vi "流量计UI.vi"() -> ()   [LabVIEW 2016]
uses:
  <vilib>/Plasmionique/MB Master/MB_Master_Serial/MB_Master_Serial.lvclass
  D:/Program Files (x86)/National Instruments/LabVIEW 2016/vi.lib/Plasmionique/MB Master/MB_Master/MB_Master.lvclass
  <vilib>/Analysis/baseanly.llb/Mean (DBL).vi
  <vilib>/Utility/config.llb/NI_LVConfig.lvlib
  <vilib>/Analysis/NI_AALBase.lvlib
panel:
  out "水位":dbl
  out "累积流量":dbl
  out "瞬时流速":dbl
  out "瞬时流量":dbl
  in  "选项卡控件":enum32{"LDM51", "MGG/KL QC", "斯坦道功率测流"}(tab)
  out "数组":T1[](array[typedef])
  out "数组 2":T2[](array[typedef]) {"累积流量单位" items=["L", "M3", "T", "USG"]; "瞬时流量单位" items=["L/S", "L/M", "L/H", "M3/S", "M3/M", "M3/H", "T/S", "T/M", "T/H", "GPS", "GPM", "GPH"]}
  out "数组 3":T5[](array[typedef])
  out "MB_Serial session":refnum<class "MB_Master_Serial.lvclass">
  in  "斯坦道功率测流":bool
  in  "流量计启用 3":bool
  in  "数量 3":u16
  out "流量计类型 3":T6=enum."斯坦道功率测流"
  in  "流量计启用 2":bool
  in  "数量 2":u16
  out "流量计类型 2":T6=enum."MGG/KL QC"
  in  "数量":u16
  out "流量计类型":T6
  in  "流量计启用":bool
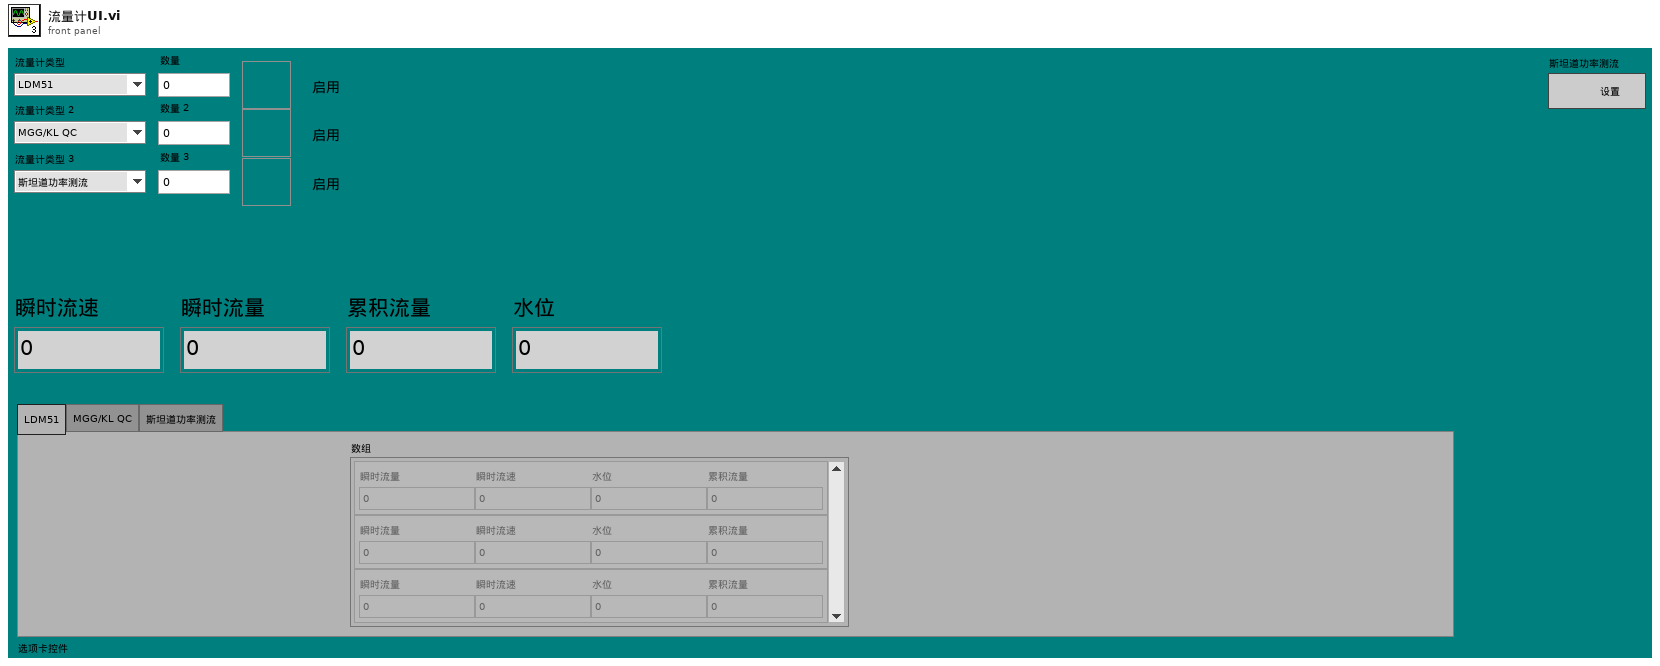
[diagram p1: front panel]
types:
  T1 = typedef "LDM51明渠流量计.lvlib/读取值.ctl" = cluster{"瞬时流量":sgl, "瞬时流速":sgl, "水位":sgl, "累积流量":sgl}
  T2 = typedef "MGG-KL-QC流量计.lvlib/读取值.ctl" = cluster{"瞬时流量":sgl, "瞬时流速":sgl, "流量百分比":sgl, "流体电导比":sgl, "正向累积数值":sgl, "反向累积数值":sgl, "瞬时流量单位":T3, "累积流量单位":T4, "上限报警":u16, "下限报警":u16, "空管报警":u16, "系统报警":u16}
  T3 = typedef "MGG-KL-QC流量计.lvlib/瞬时流量单位.ctl" = u16
  T4 = typedef "MGG-KL-QC流量计.lvlib/累积流量单位.ctl" = u16
  T5 = typedef "斯坦道功率测流.lvlib/状态值.ctl" = cluster{"1号瞬时流量":dbl, "2号瞬时流量":dbl, "3号瞬时流量":dbl, "4号瞬时流量":dbl, "5号瞬时流量":dbl, "6号瞬时流量":dbl, "1号累积流量":dbl, "2号累积流量":dbl, "3号累积流量":dbl, "4号累积流量":dbl, "5号累积流量":dbl, "6号累积流量":dbl, "总瞬时流量":dbl, "总累积流量":dbl}
  T6 = typedef "流量计类型.ctl" = enum16{"LDM51", "MGG/KL QC", "斯坦道功率测流"}
  T7 = typedef "LVDateTimeRec.ctl" = cluster{"秒数的小数部分":dbl, "秒":i32, "分":i32, "时":i32, "日":i32, "月":i32, "年":i32, "天数（周）":i32, "天数（年）":i32, "DST":i32}
  T8 = cluster{"时间标识":timestamp, "监测值":sgl, "单位":string}
  T9 = typedef "NI_LVConfig.lvlib/Config Data RefNum.ctl" = refnum<k1>
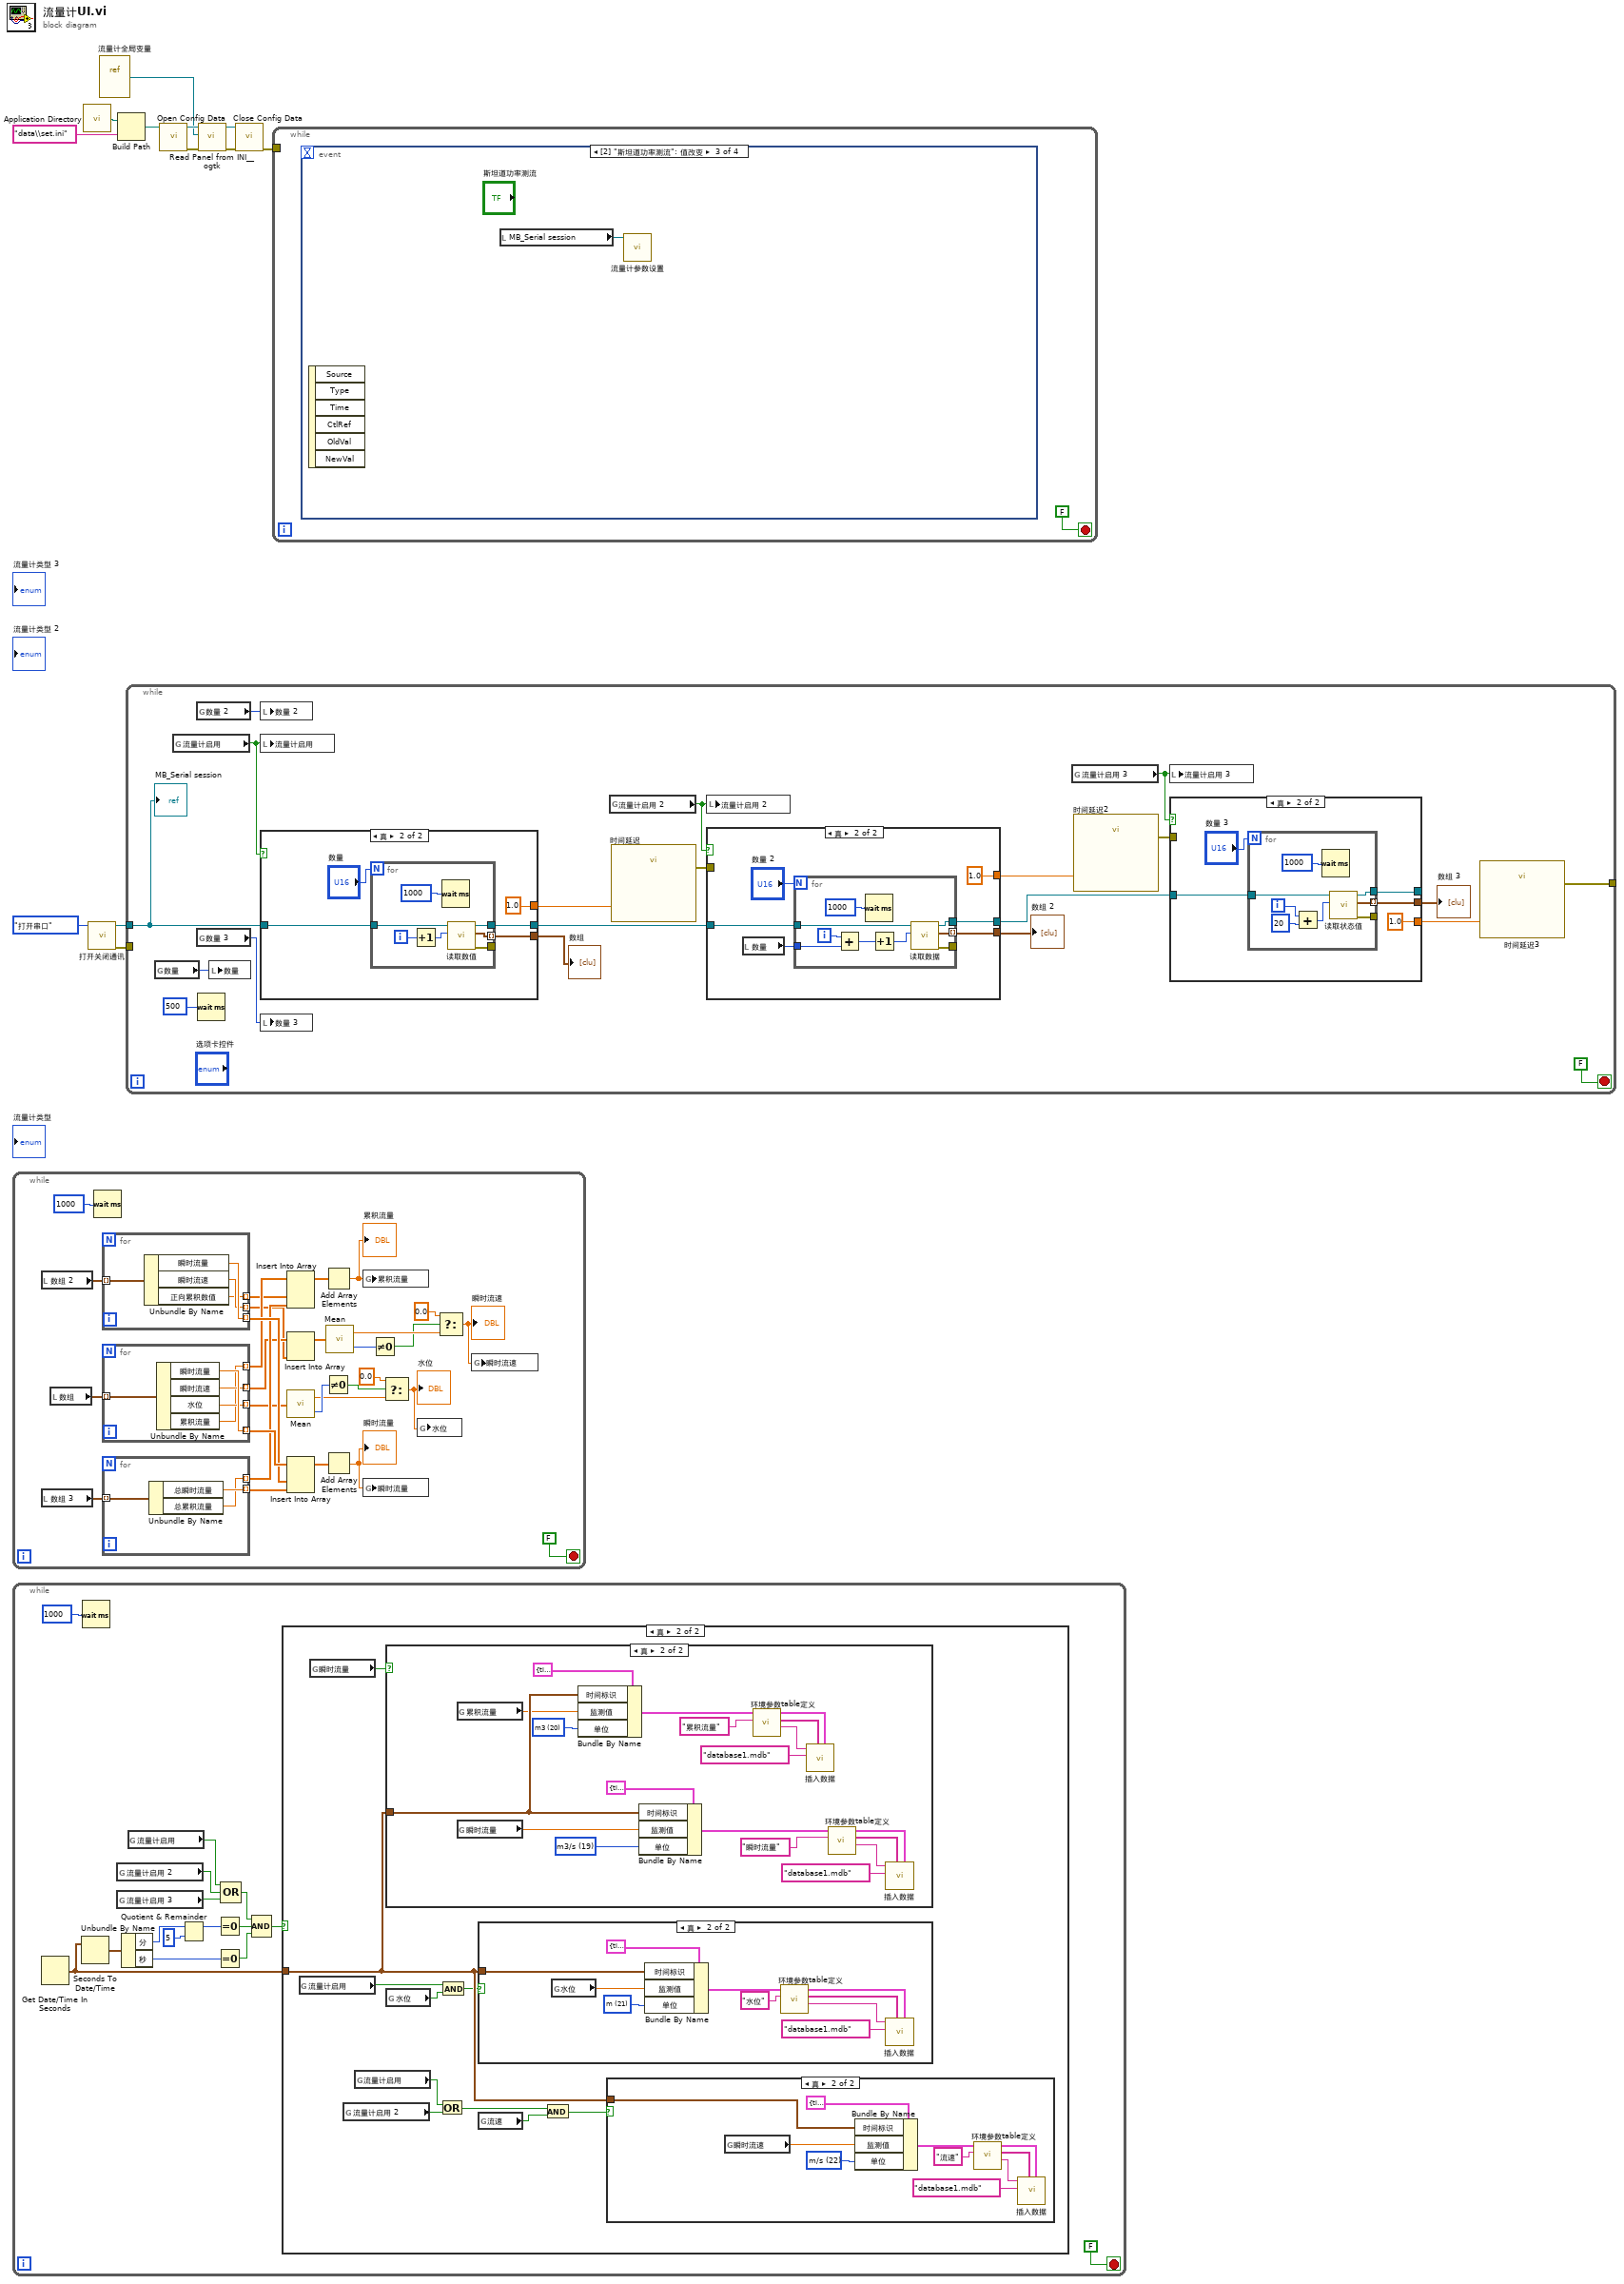
[diagram p0: block diagram]
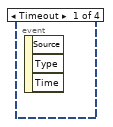
[diagram p6: hidden frame]
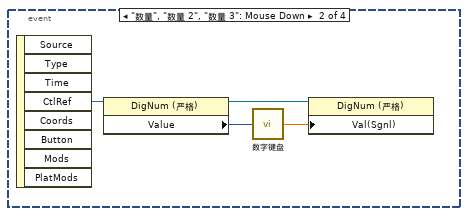
[diagram p7: hidden frame]
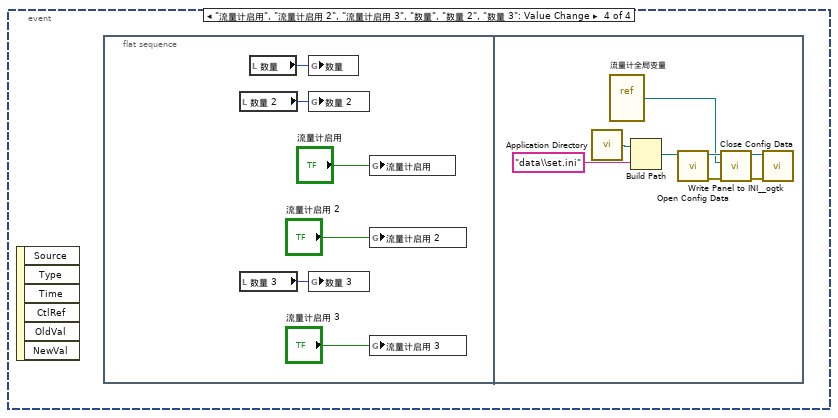
[diagram p8: hidden frame]
diagram:
  n1 = while {
    stop <- FALSE stop-if-true
    n2 = local read "数组 2"() -> (w38:T2[])
    n3 = local read "数组 3"() -> (w37:T5[])
    n4 = local read "数组"() -> (w41:T1[])
    n5 = Wait (ms)(milliseconds to wait=u32 1000 ("等待时间（毫秒）")) -> ()  [unwired: 1 out]
    n6 = for {
      tunnel: w38 -> [w48] mode=indexing
      tunnel: [w47] -> w35 mode=indexing
      tunnel: [w46] -> w27 mode=indexing
      tunnel: [w45] -> w32 mode=indexing
      n7 = Unbundle By Name(w48) -> ("瞬时流量"=w47:sgl, "瞬时流速"=w46:sgl, "正向累积数值"=w45:sgl)
    }
    n8 = for {
      tunnel: w41 -> [w53] mode=indexing
      tunnel: [w52] -> w36 mode=indexing
      tunnel: [w51] -> w28 mode=indexing
      tunnel: [w50] -> w17 mode=indexing
      tunnel: [w49] -> w33 mode=indexing
      n9 = Unbundle By Name(w53) -> ("瞬时流量"=w52:sgl, "瞬时流速"=w51:sgl, "水位"=w50:sgl, "累积流量"=w49:sgl)
    }
    n10 = for {
      tunnel: w37 -> [w44] mode=indexing
      tunnel: [w43] -> w34 mode=indexing
      tunnel: [w42] -> w31 mode=indexing
      n11 = Unbundle By Name(w44) -> ("总瞬时流量"=w43:dbl, "总累积流量"=w42:dbl)
    }
    n12 = Insert Into Array(array=w33, new element #1=w32, new element #2=w31) -> (w29:sgl[])  [unwired: 1 in]
    n13 = Insert Into Array(array=w28, new element=w27) -> (w22:sgl[])  [unwired: 1 in]
    n14 = call-poly <vilib>:"Mean.vi"("X"=w17) -> ("mean"=w18:dbl, "error"=w21:i32)
    n15 = Insert Into Array(array=w36, new element #1=w35, new element #2=w34) -> (w30:sgl[])  [unwired: 1 in]
    n16 = Add Array Elements(numeric array=w29) -> (sum=w14:sgl)
    "累积流量" <- w14
    n17 = Not Equal To 0?(x=w21) -> (x != 0?=w20:bool)
    n18 = Add Array Elements(numeric array=w30) -> (sum=w16:sgl)
    "瞬时流量" <- w16
    n19 = call-poly <vilib>:"Mean.vi"("X"=w22) -> ("mean"=w26:dbl, "error"=w23:i32)
    n20 = global write "流量计全局变量.vi" "累积流量"(w14) -> ()
    n21 = global write "流量计全局变量.vi" "瞬时流量"(w16) -> ()
    n22 = Not Equal To 0?(x=w23) -> (x != 0?=w24:bool)
    n23 = Select(t=0.0, s=w20, f=w18) -> (s? t:f=w13:dbl)
    "水位" <- w13
    n24 = global write "流量计全局变量.vi" "水位"(w13) -> ()
    n25 = Select(t=0.0, s=w24, f=w26) -> (s? t:f=w15:dbl)
    "瞬时流速" <- w15
    n26 = global write "流量计全局变量.vi" "瞬时流速"(w15) -> ()
  }
  n27 = while {
    stop <- FALSE stop-if-true
    n28 = Get Date/Time In Seconds() -> (seconds since 1Jan1904=w67:timestamp)
    n29 = Seconds To Date/Time(time stamp (now)=w67) -> (date time rec=w66:T7)  [unwired: 1 in]
    n30 = Wait (ms)(milliseconds to wait=u32 1000 ("等待时间（毫秒）")) -> ()  [unwired: 1 out]
    n31 = global read "流量计全局变量.vi" "流量计启用 2"() -> (w56:bool)
    n32 = global read "流量计全局变量.vi" "流量计启用 3"() -> (w55:bool)
    n33 = Unbundle By Name(w66) -> ("分"=w65:i32, "秒"=w63:i32)
    n34 = global read "流量计全局变量.vi" "流量计启用"() -> (w57:bool)
    n35 = Quotient & Remainder(x=w65, y=5) -> (x-y*floor(x/y)=w62:i32)  [unwired: 1 out]
    n36 = Equal To 0?(x=w62) -> (x = 0?=w61:bool)
    n37 = Equal To 0?(x=w63) -> (x = 0?=w60:bool)
    n38 = Compound Arithmetic op=OR ("复合运算")(w57, w56, w55) -> (w54:bool)
    n39 = Compound Arithmetic op=AND ("复合运算")(w54, w61, w60) -> (w59:bool)
    n40 = case shown="真" w59 {
      tunnel: w67 -> [_ w77]
      frame False {
      }
      frame True {
        n41 = global read "流量计全局变量.vi" "流量计启用"() -> (w75:bool)
        n42 = global read "副屏设置全局变量.vi" "瞬时流量"() -> (w78:bool)
        n43 = global read "流量计全局变量.vi" "流量计启用 2"() -> (w69:bool)
        n44 = global read "流量计全局变量.vi" "流量计启用"() -> (w70:bool)
        n45 = case shown="真" w78 {
          tunnel: w77 -> [_ w95]
          frame False {
          }
          frame True {
            w89 = u16 20 items=["ug/L", "mg/L", "ppm", "mg/m3", "cm", "ppb", "ug/m3", "%", "nmol/mol", "umol/mol", "MPN/L", "MPN/100ml", "ng/m3", "NTU", "无量纲", "ms/cm", "us/cm", "℃", "V", "m3/s", "m3", "m", "m/s"] ("单位")
            w91 = u16 19 items=["ug/L", "mg/L", "ppm", "mg/m3", "cm", "ppb", "ug/m3", "%", "nmol/mol", "umol/mol", "MPN/L", "MPN/100ml", "ng/m3", "NTU", "无量纲", "ms/cm", "us/cm", "℃", "V", "m3/s", "m3", "m", "m/s"] ("单位")
            n46 = global read "流量计全局变量.vi" "累积流量"() -> (w90:dbl)
            n47 = global read "流量计全局变量.vi" "瞬时流量"() -> (w92:dbl)
            n48 = Bundle By Name(cluster=cluster{"时间标识":timestamp, "监测值":sgl, "单位":u16} {"时间标识"=timestamp(0 s since 1904-01-01), "监测值"=0.0, "单位"=0} ("data"), "时间标识"=w95, "监测值"=w90, "单位"=w89) -> (w98:cluster{"时间标识":timestamp, "监测值":sgl, "单位":u16})
            n49 = Bundle By Name(cluster=cluster{"时间标识":timestamp, "监测值":sgl, "单位":u16} {"时间标识"=timestamp(0 s since 1904-01-01), "监测值"=0.0, "单位"=0} ("data"), "时间标识"=w95, "监测值"=w92, "单位"=w91) -> (w105:cluster{"时间标识":timestamp, "监测值":sgl, "单位":u16})
            n50 = call "环境参数table定义.vi"("table 输入"="累积流量", "data"=w98) -> ("table 输出"=w101:string, "columns"=w100:string[], "data输出"=w99:T8)  [unwired: 7 in]
            n51 = call "插入数据.vi"("data"=w99, "columns"=w100, "database"="database1.mdb" ("table 输入"), "table"=w101) -> ()  [unwired: 7 in, 1 out]
            n52 = call "环境参数table定义.vi"("table 输入"="瞬时流量", "data"=w105) -> ("table 输出"=w102:string, "columns"=w103:string[], "data输出"=w104:T8)  [unwired: 7 in]
            n53 = call "插入数据.vi"("data"=w104, "columns"=w103, "database"="database1.mdb" ("table 输入"), "table"=w102) -> ()  [unwired: 7 in, 1 out]
          }
        }
        n54 = global read "副屏设置全局变量.vi" "水位"() -> (w76:bool)
        n55 = Or(x=w70, y=w69) -> (x .or. y?=w71:bool)
        n56 = And(x=w75, y=w76) -> (x .and. y?=w74:bool)
        n57 = case shown="真" w74 {
          tunnel: w77 -> [_ w81]
          frame False {
          }
          frame True {
            w79 = u16 21 items=["ug/L", "mg/L", "ppm", "mg/m3", "cm", "ppb", "ug/m3", "%", "nmol/mol", "umol/mol", "MPN/L", "MPN/100ml", "ng/m3", "NTU", "无量纲", "ms/cm", "us/cm", "℃", "V", "m3/s", "m3", "m", "m/s"] ("单位")
            n58 = global read "流量计全局变量.vi" "水位"() -> (w80:dbl)
            n59 = Bundle By Name(cluster=cluster{"时间标识":timestamp, "监测值":sgl, "单位":u16} {"时间标识"=timestamp(0 s since 1904-01-01), "监测值"=0.0, "单位"=0} ("data"), "时间标识"=w81, "监测值"=w80, "单位"=w79) -> (w86:cluster{"时间标识":timestamp, "监测值":sgl, "单位":u16})
            n60 = call "环境参数table定义.vi"("table 输入"="水位", "data"=w86) -> ("table 输出"=w82:string, "columns"=w83:string[], "data输出"=w84:T8)  [unwired: 7 in]
            n61 = call "插入数据.vi"("data"=w84, "columns"=w83, "database"="database1.mdb" ("table 输入"), "table"=w82) -> ()  [unwired: 7 in, 1 out]
          }
        }
        n62 = global read "副屏设置全局变量.vi" "流速"() -> (w73:bool)
        n63 = And(x=w71, y=w73) -> (x .and. y?=w72:bool)
        n64 = case shown="真" w72 {
          tunnel: w77 -> [_ w110]
          frame False {
          }
          frame True {
            w108 = u16 22 items=["ug/L", "mg/L", "ppm", "mg/m3", "cm", "ppb", "ug/m3", "%", "nmol/mol", "umol/mol", "MPN/L", "MPN/100ml", "ng/m3", "NTU", "无量纲", "ms/cm", "us/cm", "℃", "V", "m3/s", "m3", "m", "m/s"] ("单位")
            n65 = global read "流量计全局变量.vi" "瞬时流速"() -> (w109:dbl)
            n66 = Bundle By Name(cluster=cluster{"时间标识":timestamp, "监测值":sgl, "单位":u16} {"时间标识"=timestamp(0 s since 1904-01-01), "监测值"=0.0, "单位"=0} ("data"), "时间标识"=w110, "监测值"=w109, "单位"=w108) -> (w115:cluster{"时间标识":timestamp, "监测值":sgl, "单位":u16})
            n67 = call "环境参数table定义.vi"("table 输入"="流速", "data"=w115) -> ("table 输出"=w111:string, "columns"=w112:string[], "data输出"=w113:T8)  [unwired: 7 in]
            n68 = call "插入数据.vi"("data"=w113, "columns"=w112, "database"="database1.mdb" ("table 输入"), "table"=w111) -> ()  [unwired: 7 in, 1 out]
          }
        }
      }
    }
  }
  n69 = call <vilib>:"Application Directory.vi"() -> ("Application Directory"=w10:path)
  n70 = call "打开关闭通讯.vi"("功能输入"=enum16{"打开串口", "关闭串口"}."打开串口") -> ("error out"=w3:errorcluster, "MB_Serial session"=w2:refnum<class "MB_Master_Serial.lvclass">)  [unwired: 9 in]
  n71 = vi-ref "流量计全局变量.vi"() -> (w1:refnum<vi>)
  n72 = Build Path(base path=w10, name or relative path="data\\set.ini" ("名称或相对路径")) -> (appended path=w11:path)
  n73 = while {
    tunnel: w3 -> [_]
    tunnel: w2 -> [w127]
    tunnel: [w118] -> _
    stop <- FALSE stop-if-true
    n74 = global read "流量计全局变量.vi" "数量"() -> (w126:u16)
    n75 = global read "流量计全局变量.vi" "流量计启用"() -> (w135:bool)
    n76 = global read "流量计全局变量.vi" "数量 2"() -> (w125:u16)
    n77 = global read "流量计全局变量.vi" "数量 3"() -> (w124:u16)
    n78 = Wait (ms)(milliseconds to wait=u32 500 ("等待时间（毫秒）")) -> ()  [unwired: 1 out]
    n79 = local write "数量"(w126) -> ()
    n80 = local write "数量 2"(w125) -> ()
    n81 = local write "流量计启用"(w135) -> ()
    n82 = case shown="真" w135 {
      tunnel: w127 -> [w168 w173]
      tunnel: [w168 w171] -> w134
      tunnel: [_ w170] -> w132
      tunnel: [_ 1.0 ("Delay Time (s)")] -> w123
      frame False {
      }
      frame True {
        n83 = for {
          N: "数量" -> [_]
          tunnel: w173 -> [w180]
          tunnel: [w179] -> _
          tunnel: [w176] -> w171
          tunnel: [w175] -> w170 mode=indexing
          i -> [w178]
          n84 = Increment(x=w178) -> (x+1=w177:i32)
          n85 = Wait (ms)(milliseconds to wait=u32 1000 ("等待时间（毫秒）")) -> ()  [unwired: 1 out]
          n86 = call "读取数值.vi"("Slave ID"=w177, "MB session in"=w180) -> ("error out"=w179:errorcluster, "读取值"=w175:T1, "MB session out"=w176:refnum<class "MB_Master_Serial.lvclass">)  [unwired: 7 in]
        }
      }
    }
    "数组" <- w132
    n87 = local write "数量 3"(w124) -> ()
    n88 = global read "流量计全局变量.vi" "流量计启用 2"() -> (w133:bool)
    n89 = call "时间延迟"("Delay Time (s)"=w123) -> ("error out"=w122:errorcluster)  [unwired: 10 in]
    n90 = local write "流量计启用 2"(w133) -> ()
    n91 = case shown="真" w133 {
      tunnel: w134 -> [w152 w157]
      tunnel: [w152 w155] -> w130
      tunnel: [_ w154] -> w131
      tunnel: w122 -> [_ _]
      tunnel: [_ 1.0 ("Delay Time (s)")] -> w121
      frame False {
      }
      frame True {
        n92 = local read "数量"() -> (w156:u16)
        n93 = for {
          N: "数量 2" -> [_]
          tunnel: w157 -> [w166]
          tunnel: w156 -> [w163]
          tunnel: [w162] -> w155
          tunnel: [w161] -> w154 mode=indexing
          tunnel: [w160] -> _
          i -> [w164]
          n94 = Add(x=w164, y=w163) -> (x+y=w165:i32)
          n95 = Wait (ms)(milliseconds to wait=u32 1000 ("等待时间（毫秒）")) -> ()  [unwired: 1 out]
          n96 = Increment(x=w165) -> (x+1=w167:i32)
          n97 = call "读取数据.vi"("Slave ID"=w167, "MB session in"=w166) -> ("error out"=w160:errorcluster, "读取值"=w161:T2, "MB session out"=w162:refnum<class "MB_Master_Serial.lvclass">)  [unwired: 6 in, 1 out]
        }
      }
    }
    "数组 2" <- w131
    n98 = global read "流量计全局变量.vi" "流量计启用 3"() -> (w129:bool)
    n99 = call "时间延迟2"("Delay Time (s)"=w121) -> ("error out"=w119:errorcluster)  [unwired: 10 in]
    n100 = local write "流量计启用 3"(w129) -> ()
    n101 = case shown="真" w129 {
      tunnel: w130 -> [w138 w143]
      tunnel: [w138 w142] -> _
      tunnel: [_ w140] -> w128
      tunnel: [_ 1.0 ("Delay Time (s)")] -> w120
      tunnel: w119 -> [_ _]
      frame False {
      }
      frame True {
        n102 = for {
          N: "数量 3" -> [_]
          tunnel: w143 -> [w149]
          tunnel: [w146] -> w142
          tunnel: [w147] -> _
          tunnel: [w145] -> w140 mode=indexing
          i -> [w151]
          n103 = Add(x=w151, y=20) -> (x+y=w148:i32)
          n104 = Wait (ms)(milliseconds to wait=u32 1000 ("等待时间（毫秒）")) -> ()  [unwired: 1 out]
          n105 = call "读取状态值.vi"("Slave ID"=w148, "MB session in"=w149) -> ("error out"=w147:errorcluster, "状态值"=w145:T5, "MB session out"=w146:refnum<class "MB_Master_Serial.lvclass">)  [unwired: 6 in, 1 out]
        }
      }
    }
    "数组 3" <- w128
    n106 = call "时间延迟3"("Delay Time (s)"=w120) -> ("error out"=w118:errorcluster)  [unwired: 10 in]
    "MB_Serial session" <- w127
  }
  n107 = call <vilib>:"Open Config Data.vi"("configuration file path"=w11) -> ("error out"=w8:errorcluster, "refnum"=w9:T9)  [unwired: 8 in, 1 out]
  n108 = call <userlib>:"Read Panel from INI__ogtk.vi"("error in (no error)"=w8, "VI ref"=w1, "refnum"=w9) -> ("error out"=w6:errorcluster, "refnum out"=w7:T9)  [unwired: 7 in]
  n109 = call <vilib>:"Close Config Data.vi"("error in (no error)"=w6, "refnum"=w7) -> ("error out"=w5:errorcluster)  [unwired: 8 in, 1 out]
  n110 = while {
    tunnel: w5 -> [_]
    stop <- FALSE stop-if-true
    n111 = event shown="[2] \"斯坦道功率测流\": 值改变" {
      selector: _ -> [_ _ _ _]
      dyn-events: _ -> [_ _ _ _]
      timeout: _ -> [_ _ _ _]
      event Timeout {
        n112 = event-data() -> ()  [unwired: 1 in, 3 out]
      }
      event "数量", "数量 2", "数量 3": Mouse Down {
        n113 = event-data() -> ("CtlRef"=w185:refnum<vi>)  [unwired: 1 in, 7 out]
        n114 = property class="DigNum (严格)"(reference=w185) -> (reference out=w183:refnum<vi>, "Value"=w184:u16)  [unwired: 1 in, 1 out]
        n115 = call "数字键盘.vi"("OldNumber"=w184) -> ("NewNumber"=w182:sgl)
        n116 = property class="DigNum (严格)"(reference=w183, "Val(Sgnl)"=w182) -> ()  [unwired: 1 in, 2 out]
      }
      event "斯坦道功率测流": Value Change {
        n117 = event-data() -> ()  [unwired: 1 in, 6 out]
        n118 = local read "MB_Serial session"() -> (w186:refnum<class "MB_Master_Serial.lvclass">)
        n119 = call "流量计参数设置.vi"("MB session in"=w186) -> ()  [unwired: 11 in]
      }
      event "流量计启用", "流量计启用 2", "流量计启用 3", "数量", "数量 2", "数量 3": Value Change {
        n120 = event-data() -> ()  [unwired: 1 in, 6 out]
        n121 = flat-sequence {
          frame #0 {
            n122 = local read "数量 2"() -> (w188:u16)
            n123 = local read "数量 3"() -> (w187:u16)
            n124 = local read "数量"() -> (w189:u16)
            n125 = global write "流量计全局变量.vi" "数量"(w189) -> ()
            n126 = global write "流量计全局变量.vi" "数量 2"(w188) -> ()
            n127 = global write "流量计全局变量.vi" "数量 3"(w187) -> ()
            n128 = global write "流量计全局变量.vi" "流量计启用"("流量计启用") -> ()
            n129 = global write "流量计全局变量.vi" "流量计启用 2"("流量计启用 2") -> ()
            n130 = global write "流量计全局变量.vi" "流量计启用 3"("流量计启用 3") -> ()
          }
          frame #1 {
            n131 = call <vilib>:"Application Directory.vi"() -> ("Application Directory"=w196:path)
            n132 = vi-ref "流量计全局变量.vi"() -> (w193:refnum<vi>)
            n133 = Build Path(base path=w196, name or relative path="data\\set.ini" ("名称或相对路径")) -> (appended path=w195:path)
            n134 = call <vilib>:"Open Config Data.vi"("configuration file path"=w195) -> ("error out"=w198:errorcluster, "refnum"=w200:T9)  [unwired: 8 in, 1 out]
            n135 = call <userlib>:"Write Panel to INI__ogtk.vi"("error in (no error)"=w198, "VI ref"=w193, "refnum"=w200) -> ("error out"=w197:errorcluster, "refnum out"=w199:T9)  [unwired: 7 in]
            n136 = call <vilib>:"Close Config Data.vi"("error in (no error)"=w197, "refnum"=w199) -> ()  [unwired: 8 in, 2 out]
          }
        }
      }
    }
  }
